vi "Initialize.vi"(8 "error in (no error)":errorcluster, 11 "VICI Settings":T1 {"Pump Number" min=0.0 max=20.0 step=1.0}) -> (0 "error out":errorcluster, 1 "Initialized":bool, 2 "No Pump Connected":bool, 3 "VICI Settings":T1 {"Pump Number" min=0.0 max=20.0 step=1.0})   [LabVIEW 2018, in "VICI M50.lvlib"]
uses:
  VICI M50.lvlib
  Settings Cluster.ctl
  <vilib>/Instr/_visa.llb/VISA Configure Serial Port (Instr).vi
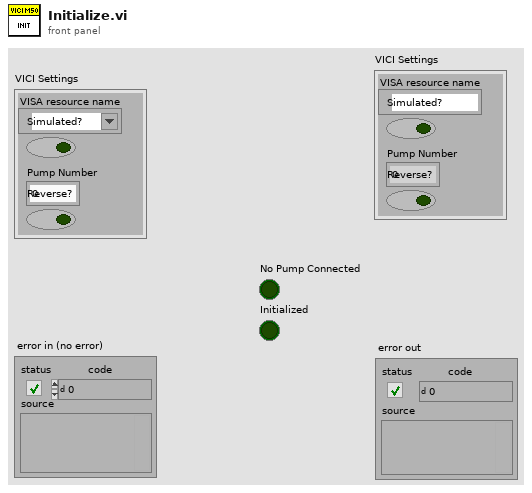
[diagram p1: front panel]
types:
  T1 = typedef "VICI M50.lvlib/Settings Cluster.ctl" = cluster{"VISA resource name":refnum<visa-resource-name>, "Simulated?":bool, "Pump Number":dbl, "Reverse?":bool}
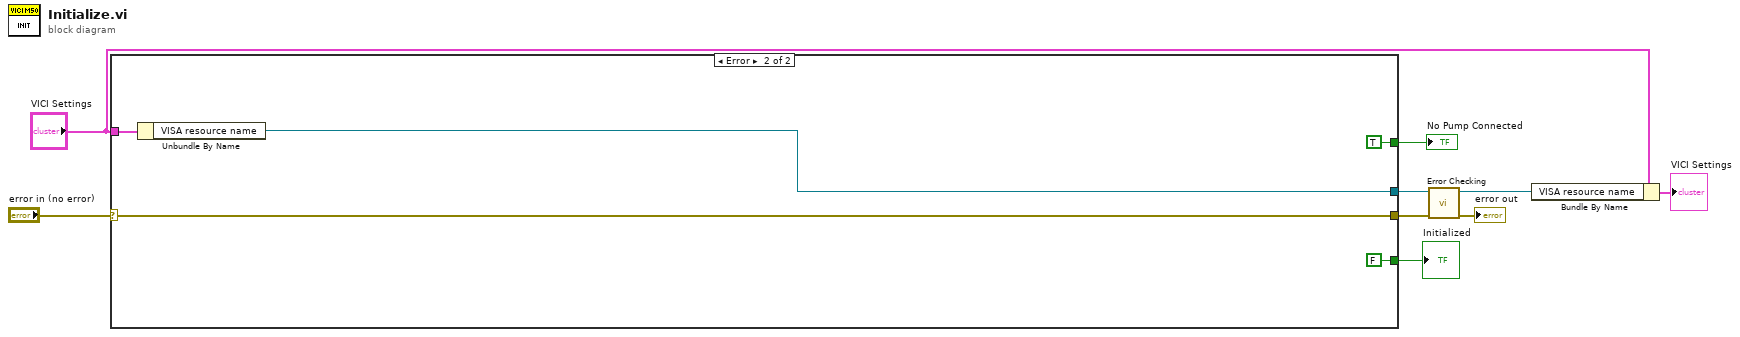
[diagram p0: block diagram]
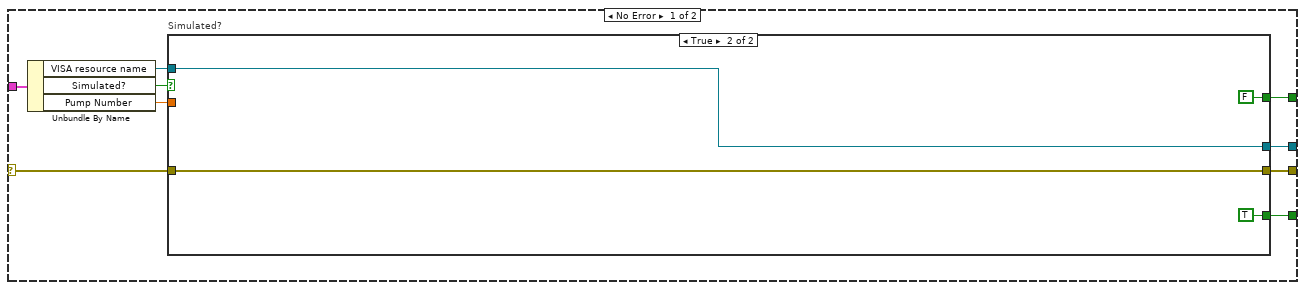
[diagram p2: hidden frame]
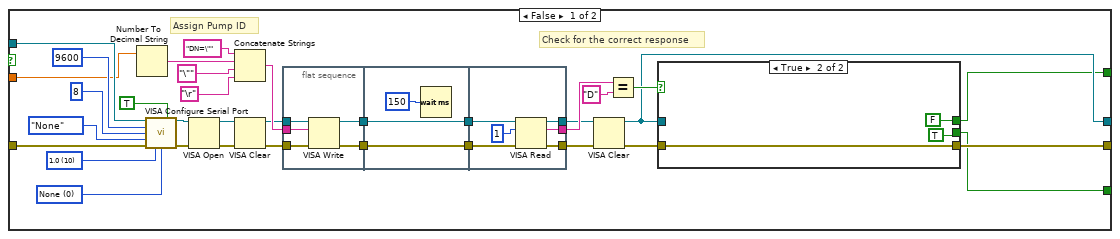
[diagram p3: hidden frame]
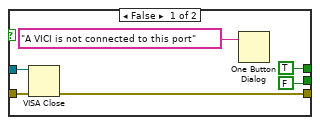
[diagram p4: hidden frame]
diagram:
  n1 = case shown="Error" "error in (no error)" {
    selector: "error in (no error)" -> [w18 w84]
    tunnel: "VICI Settings" -> [w15 w83]
    tunnel: [w16 w84] -> w5
    tunnel: [w13 w82] -> w6
    tunnel: [w11 FALSE] -> w2
    tunnel: [w10 TRUE] -> w1
    frame No Error {
      n2 = Unbundle By Name(w15) -> ("VISA resource name"=w14:refnum<visa-resource-name>, "Simulated?"=w17:bool, "Pump Number"=w12:dbl)
      n3 = case "Simulated?" shown="True" w17 {
        tunnel: w18 -> [w46 w79]
        tunnel: [w21 w79] -> w16
        tunnel: [w28 w78] -> w13
        tunnel: w14 -> [w44 w78]
        tunnel: w12 -> [w39 _]
        tunnel: [w20 TRUE] -> w11
        tunnel: [w19 FALSE] -> w10
        frame False {
          w48 = u16 0 items=["None", "XON/XOFF", "RTS/CTS", "XON/XOFF & RTS/CTS", "DTR/DSR", "XON/XOFF & DTR/DSR"] ("flow control (0:none)")
          w49 = u16 10 items=["1.0"=10, "1.5"=15, "2.0"=20] ("stop bits (10: 1 bit)")
          # "Check for the correct response"
          # "Assign Pump ID"
          n4 = Number To Decimal String(number=w39) -> (decimal integer string=w40:string)  [unwired: 1 in]
          n5 = call-poly "VISA Configure Serial Port"("VISA resource name"=w44, "Enable Termination\nChar (T)"=TRUE ("Enable Termination\nChar (T)"), "baud rate (9600)"=u32 9600, "data bits (8)"=u16 8, "parity (0:none)"=enum16{"None", "Odd", "Even", "Mark", "Space"}."None", "error in (no error)"=w46, "stop bits (10: 1 bit)"=w49, "flow control (0:none)"=w48) -> ("VISA resource name out"=w45:refnum<visa-resource-name>, "error out"=w47:errorcluster)  [unwired: 6 in]
          n6 = VISA Open(error in (no error)=w47, VISA resource name=w45) -> (VISA resource name=w27:refnum<visa-resource-name>, error out=w24:errorcluster)  [unwired: 3 in]
          n7 = Concatenate Strings("DN=\"" ("string"), w40, "\"" ("string"), "\r") -> (w36:string)
          n8 = VISA Clear(VISA resource name=w27, error in (no error)=w24) -> (VISA resource name out=w26:refnum<visa-resource-name>, error out=w25:errorcluster)
          n9 = flat-sequence {
            tunnel: w36 -> [w57]
            tunnel: [w56] -> w33
            tunnel: [w55] -> w32
            tunnel: w26 -> [w54]
            tunnel: w25 -> [w53]
            tunnel: [w59] -> w34
            tunnel: w33 -> [w59]
            tunnel: w32 -> [w58]
            tunnel: [w58] -> w31
            tunnel: [w66] -> w29
            tunnel: [w65] -> w35
            tunnel: [w64] -> w30
            tunnel: w34 -> [w62]
            tunnel: w31 -> [w61]
            frame #0 {
              n10 = VISA Write(VISA resource name=w54, write buffer=w57, error in (no error)=w53) -> (VISA resource name out=w56:refnum<visa-resource-name>, error out=w55:errorcluster)  [unwired: 1 out]
            }
            frame #1 {
              n11 = Wait (ms)(milliseconds to wait=u32 150) -> ()  [unwired: 1 out]
            }
            frame #2 {
              n12 = VISA Read(VISA resource name=w62, byte count=u32 1, error in (no error)=w61) -> (VISA resource name out=w64:refnum<visa-resource-name>, read buffer=w65:string, error out=w66:errorcluster)  [unwired: 1 out]
            }
          }
          n13 = VISA Clear(VISA resource name=w30, error in (no error)=w29) -> (VISA resource name out=w28:refnum<visa-resource-name>, error out=w22:errorcluster)
          n14 = Equal?(x=w35, y="D") -> (x = y?=w37:bool)
          n15 = case shown="True" w37 {
            tunnel: w28 -> [w71 _]
            tunnel: w22 -> [w70 w74]
            tunnel: [TRUE FALSE] -> w19
            tunnel: [w68 w74] -> w21
            tunnel: [FALSE TRUE] -> w20
            frame False {
              n16 = VISA Close(VISA resource name=w71, error in (no error)=w70) -> (error out=w68:errorcluster)
              n17 = One Button Dialog(message="A VICI is not connected to this port") -> ()  [unwired: 1 in, 1 out]
            }
            frame True {
            }
          }
        }
        frame True {
        }
      }
    }
    frame Error {
      n18 = Unbundle By Name(w83) -> ("VISA resource name"=w82:refnum<visa-resource-name>)
    }
  }
  "Initialized" <- w2
  "No Pump Connected" <- w1
  n19 = call "Error Checking.vi"("error in (no error)"=w5, "VISA resource name"=w6) -> ("error out"=→"error out":errorcluster, "VISA resource name"=w3:refnum<visa-resource-name>)  [unwired: 7 in, 1 out]
  n20 = Bundle By Name(cluster="VICI Settings", "VISA resource name"=w3) -> (→"VICI Settings":T1)
